vi "Read Source Account.vi"(8 "error in (no error)":errorcluster, 11 "ATransfer in":refnum<class "ATransfer.lvclass">) -> (0 "error out":errorcluster, 2 "Source Account":string, 3 "ATransfer out":refnum<class "ATransfer.lvclass">)   [LabVIEW 2020, in "ATransfer.lvclass"]
uses:
  ATransfer.lvclass
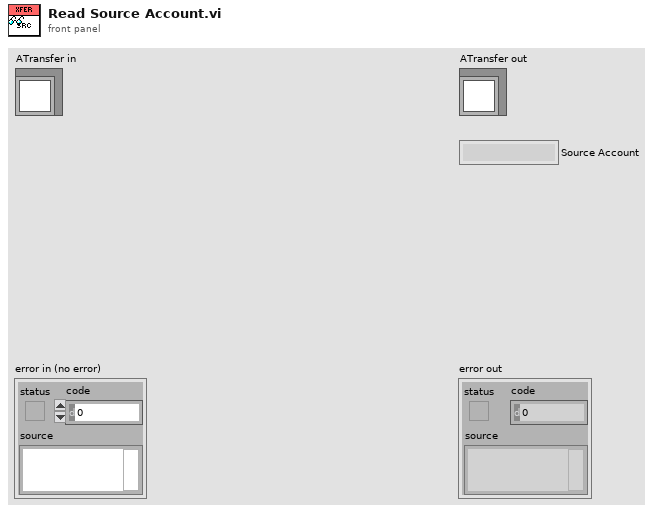
[diagram p1: front panel]
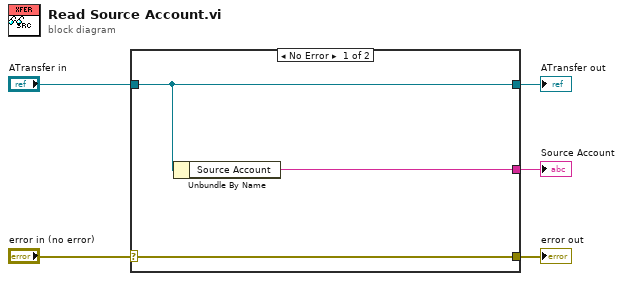
[diagram p0: block diagram]
diagram:
  n1 = case shown="No Error" "error in (no error)" {
    selector: "error in (no error)" -> [w8 w9]
    tunnel: [w8 w9] -> w4
    tunnel: [w7 w10] -> w2
    tunnel: "ATransfer in" -> [w7 w10]
    tunnel: [w6 _] -> w1
    frame No Error {
      n2 = Unbundle By Name(w7) -> ("Source Account"=w6:string)
    }
    frame Error {
    }
  }
  "error out" <- w4
  "ATransfer out" <- w2
  "Source Account" <- w1
